vi "only_serial.vi"() -> ()   [LabVIEW 2019]
uses:
  <vilib>/Platform/TimedLoop/XDataNode/timing_clust.ctl
  <vilib>/Platform/TimedLoop/XDataNode/nitl_modes.ctl
  <vilib>/Platform/TimedLoop/XDataNode/wakeup.ctl
  <vilib>/myRIO/Instrument Drivers/Onboard IO/UART/typedef/VISA Configuration.ctl
  <vilib>/FPGAPlugInAG/myRIO-1900/niLvFpga_Open_myRIO-1900.vi
  <vilib>/rvi/interface/common/dynamic/niFpgaDynamicAddResources.vi
  <vilib>/Utility/error.llb/Error Cluster From Error Code.vi
  <vilib>/rvi/errors/niLvFpgaAdjustHostInterfaceError.vi
  <vilib>/FPGAPlugInAG/Dynamic/niLvFpga_Close_Dynamic.vi
  <vilib>/Platform/TimedLoop/XDataNode/XDataNode.xnode
  <vilib>/rvi/interface/nirviOpenFPGA/nirviOpenFPGA.xnode
  FPGA Bitfiles/capstone_FPGATarget_encoderFPGA_AeXAVEDpCcY.lvbitx
  encoder_FPGA.vi
  <vilib>/rvi/interface/nirviReadWriteControl/nirviReadWriteControl.xnode
  <vilib>/rvi/interface/nirviCloseFPGA/nirviCloseFPGA.xnode
  <vilib>/Platform/TimedLoop/XDataNode/XDNodeRunTimeDep.lvlib
  NiFpgaLv.dll
  <vilib>/rvi/interface/Simulation/niFpgaSimulationCallBeginRW.vi
  <vilib>/myRIO/Instrument Drivers/Onboard IO/UART/UART.lvlib
panel:
  in  "timed 정지":bool
  out "신중버튼 i":i32
  out "read buffer":string
  out "2번(거리)":string
  out "1번(각도)":string
  out "불리언":bool
  out "s? t:f":dbl
  in  "error in (no error)":errorcluster
  out "error out":errorcluster
  out "1or0이 들어옴":string
  out "회전수 i":i32
  in  "신중버튼":bool
  out "x > y?":bool
  in  "L_pwm":i32=3000
  out "타임아웃":i32=-1
  in  "R_pwm":i32=3000
  out "L_encoder":i32
  out "R_Encoder":i32
  out "L_이동 거리":dbl
  out "R_이동 거리":dbl
  out "mm/ms":dbl
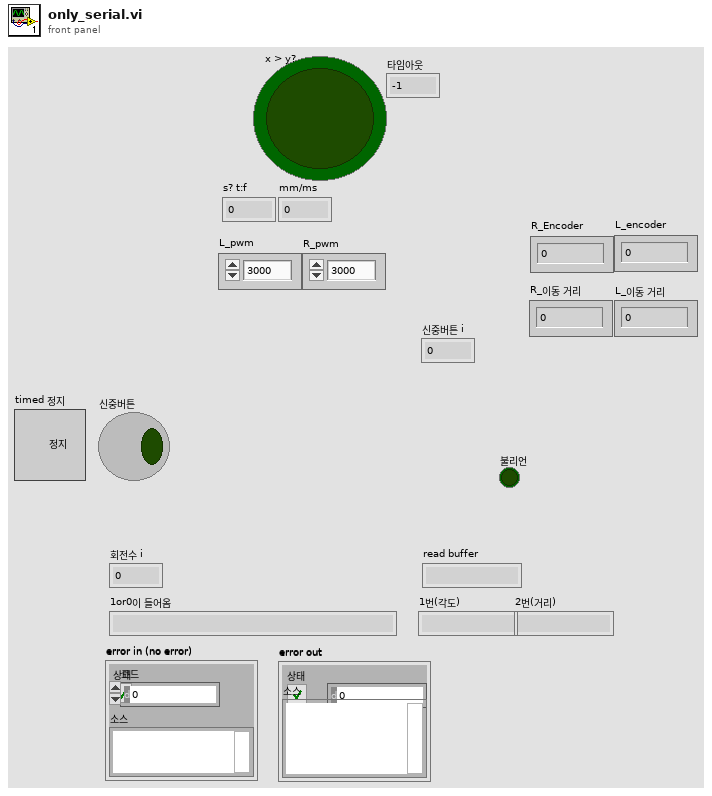
[diagram p1: front panel]
types:
  T1 = typedef "XDNodeRunTimeDep.lvlib/timing_clust.ctl" = cluster{"Expected End [f-1]":u64, "Actual End [f-1]":u64, "Finished Late? [f-1]":bool, "Expected End [i-1]":u64, "Actual End [i-1]":u64, "Finished Late? [i-1]":bool, "Expected Start [i]":u64, "Actual Start [i]":u64, "Expected Start [f]":u64, "Actual Start [f]":u64, "Source Name":string, "Structure Name":string, "Period":i64, "Deadline":i64, "Offset":i64, "Start":i64, "Priority":i32, "Timeout":i32, "Mode":T2, "Wakeup Reason":T3, "Error":errorcluster, "Source Type":string, "Secondary Source Type":string, "Global End Time":u64, "Global Start Time":u64, "Frame Duration":u64, "Iteration Duration":u64, "Assigned CPU":i32, "I/O Scan Engine Mode":u32}
  T2 = typedef "XDNodeRunTimeDep.lvlib/nitl_modes.ctl" = enum32{"No Change", "Process missed periods, maintain original phase", "Discard missed periods, maintain original phase", "Process missed periods, ignore original phase", "Discard missed periods, ignore original phase"}
  T3 = typedef "XDNodeRunTimeDep.lvlib/wakeup.ctl" = enum32{"Normal", "Aborted", "Asynchronous wakeup", "Timing source error", "Timed loop error", "Timeout"}
  T4 = typedef "UART.lvlib/VISA Configuration.ctl" = cluster{"baud rate (9600)":u32, "data bits (8)":u16, "parity (0:none)":enum16{"None", "Odd", "Even", "Mark", "Space"}, "stop bits (10: 1 bit)":u16, "flow control (0:none)":u16, "termination char\n(0xA = '\\n' = LF) ":u8, "Enable Termination\nChar (T)":bool, "timeout (10sec)":u32}
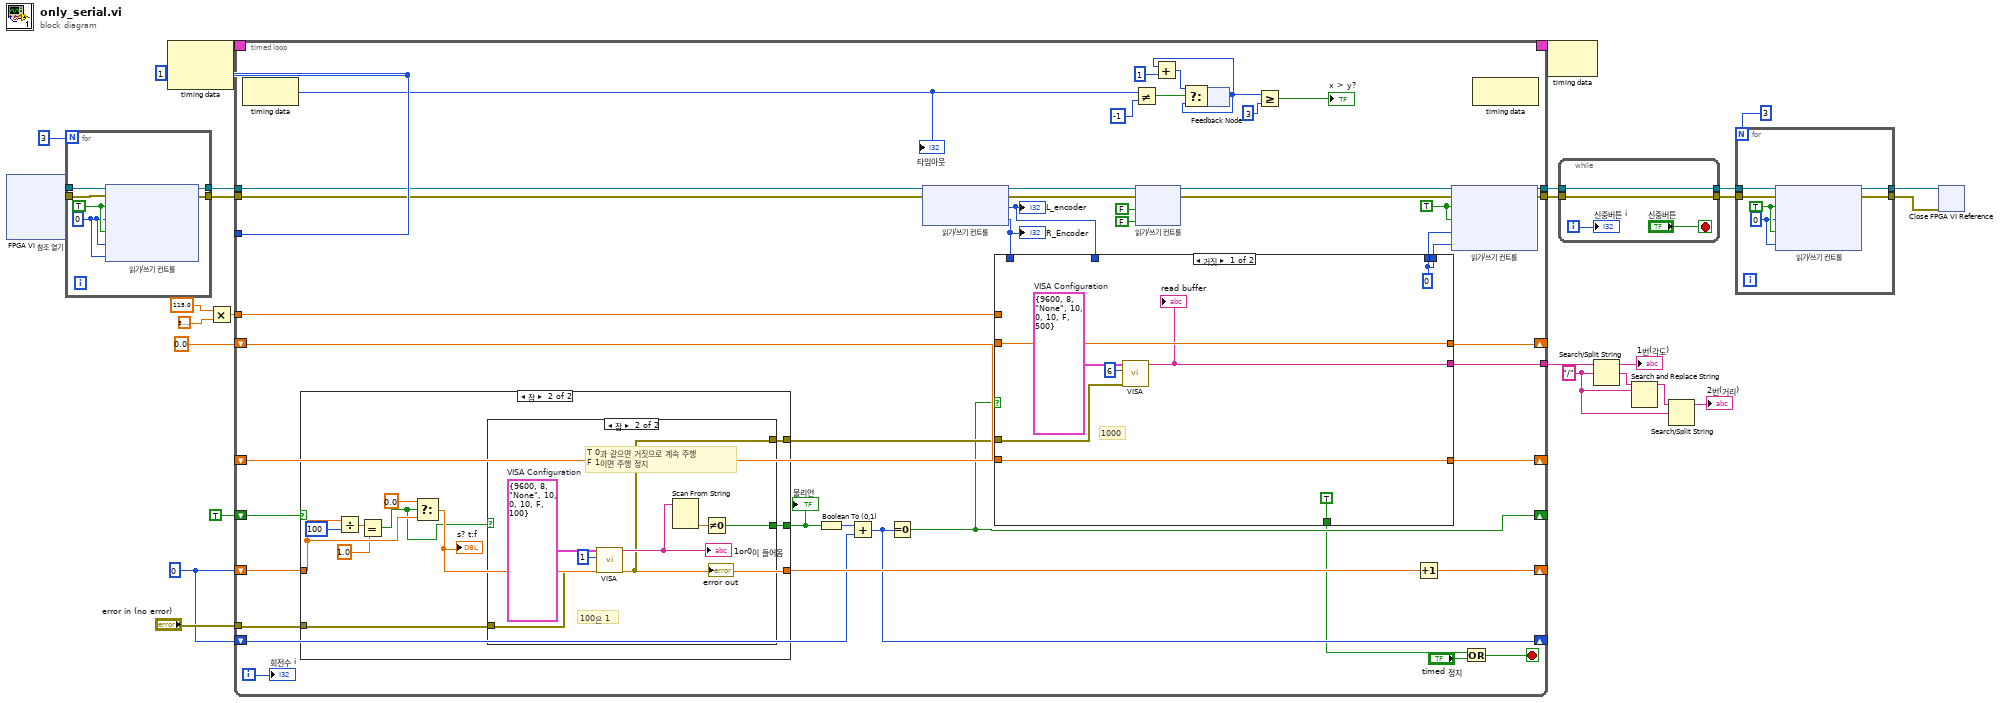
[diagram p0: block diagram]
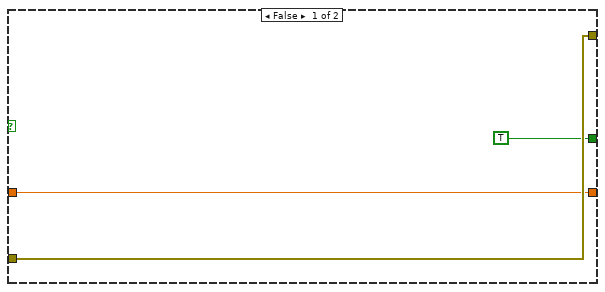
[diagram p2: hidden frame]
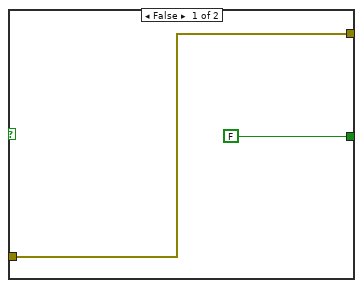
[diagram p3: hidden frame]
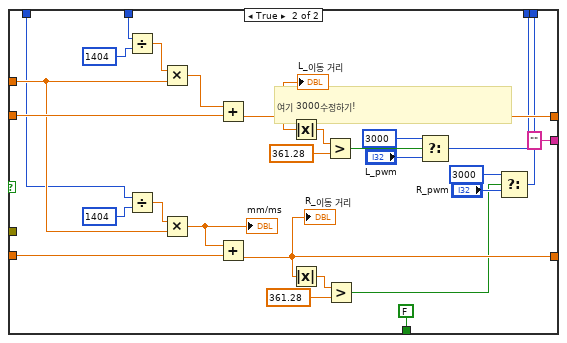
[diagram p4: hidden frame]
diagram:
  w10 = "/" ("검색 문자열/문자 (-)")
  w12 = 0
  w18 = 0.0
  w19 = i64 1 ("주기")
  n1 = xnode "FPGA VI 참조 열기"() -> ("FPGA VI 참조 출력"=w17:refnum<k20>, "에러 출력"=w16:errorcluster)  [unwired: 2 in]
  n2 = for {
    N: 3 -> [_]
    tunnel: [w34] -> w25
    tunnel: [w33] -> w24
    tunnel: w17 -> [w30]
    tunnel: w16 -> [w29]
    w31 = 0 ("pwm input(escon)")
    w32 = TRUE ("encoder reset")
    n3 = xnode "읽기/쓰기 컨트롤"("FPGA VI 참조 입력"=w30, "에러 입력"=w29, "encoder reset"=w32, "pwm input"=w31, "R_encoder reset"=w32, "R_pwm input"=w31, "직동_pwm input"=w31) -> ("FPGA VI 참조 출력"=w34:refnum<k20>, "에러 출력"=w33:errorcluster)
  }
  n4 = node-c288(w19) -> (w28:T1)  [unwired: 1 in]
  n5 = Multiply(x=115.0, y=3.141592653589793) -> (x*y=w20:dbl)
  n6 = timed-loop {
    timing: w28 -> [_]
    timing-out: [_] -> w27
    tunnel: w25 -> [w67]
    tunnel: w24 -> [w66]
    tunnel: [w70] -> w4
    tunnel: [w69] -> w1
    tunnel: w20 -> [w58]
    tunnel: w19 -> [_]
    shift-right: [w61] -> _
    shift-left: w18 -> [w59]
    shift-right: [w51] -> _
    shift-left: w18 -> [w60]
    tunnel: "error in (no error)" -> [w49]
    shift-right: [w48] -> _
    shift-left: w12 -> [w46]
    shift-right: [w42] -> _
    shift-left: w12 -> [w43]
    shift-right: [w39] -> _
    shift-left: TRUE -> [w40]
    tunnel: [w38] -> w6
    i -> [w50]
    stop <- w37 stop-if-true
    w68 = TRUE ("encoder reset")
    n7 = node-c288() -> (w79:i32)  [unwired: 1 in]
    "타임아웃" <- w79
    n8 = case shown="참" w40 {
      tunnel: w49 -> [w82 w92]
      tunnel: [w80 w90] -> w47
      tunnel: w46 -> [w80 w88]
      tunnel: [TRUE w84] -> w44
      tunnel: [w82 w83] -> w41
      frame False {
      }
      frame True {
        n9 = Divide(x=w88, y=100) -> (x/y=w87:dbl)
        n10 = Equal?(x=w87, y=1.0) -> (x = y?=w85:bool)
        n11 = Select(t=0.0, s=w85, f=w88) -> (s? t:f=w90:dbl)
        "s? t:f" <- w90
        n12 = case shown="참" w85 {
          tunnel: w92 -> [w93 w101]
          tunnel: [FALSE w100] -> w84
          tunnel: [w93 w95] -> w83
          frame False {
          }
          frame True {
            w98 = T4 {"baud rate (9600)"=9600, "data bits (8)"=8, "parity (0:none)"=enum."None", "stop bits (10: 1 bit)"=10, "flow control (0:none)"=0, "termination char\n(0xA = '\\n' = LF) "=10, "Enable Termination\nChar (T)"=FALSE, "timeout (10sec)"=100}  # VISA Configuration
            # "100은 1"
            # "T 0과 같으면 거짓으로 계속 주행\nF 1이면 주행 정지"
            n13 = call "VISA.vi"("에러 입력(에러 없음)"=w101, "바이트 카운트"=u32 1, "VISA Configuration"=w98) -> ("에러 출력"=w95:errorcluster, "read buffer"=w96:string)  [unwired: 7 in]
            "error out" <- w95
            "1or0이 들어옴" <- w96
            n14 = Scan From String(input string=w96) -> (output 1=w99:dbl)  [unwired: 4 in, 3 out]
            n15 = Not Equal To 0?(x=w99) -> (x != 0?=w100:bool)
          }
        }
      }
    }
    "불리언" <- w44
    n16 = Boolean To (0,1)(Boolean=w44) -> (0, 1=w45:i16)
    n17 = Add(x=w45, y=w43) -> (x+y=w42:i32)
    n18 = Equal To 0?(x=w42) -> (x = 0?=w39:bool)
    n19 = xnode "읽기/쓰기 컨트롤"("FPGA VI 참조 입력"=w67, "에러 입력"=w66) -> ("FPGA VI 참조 출력"=w64:refnum<k20>, "에러 출력"=w63:errorcluster, "Encoder  (4x)"=w57:i32, "R_Encoder  (4x)"=w56:i32)
    "L_encoder" <- w57
    "R_Encoder" <- w56
    n20 = case shown="거짓" w39 {
      tunnel: [w106 w136] -> w61
      tunnel: w60 -> [w107 w135]
      tunnel: w59 -> [w106 w134]
      tunnel: w58 -> [_ w133]
      tunnel: w57 -> [_ w132]
      tunnel: w56 -> [_ w131]
      tunnel: [TRUE FALSE] -> w36
      tunnel: [w109 w119] -> w53
      tunnel: [w109 w114] -> w52
      tunnel: [w107 w113] -> w51
      tunnel: w41 -> [w103 _]
      tunnel: [w102 "" ("read buffer")] -> w38
      frame False {
        w105 = T4 {"baud rate (9600)"=9600, "data bits (8)"=8, "parity (0:none)"=enum."None", "stop bits (10: 1 bit)"=10, "flow control (0:none)"=0, "termination char\n(0xA = '\\n' = LF) "=10, "Enable Termination\nChar (T)"=FALSE, "timeout (10sec)"=500}  # VISA Configuration
        w109 = 0 ("L_pwm")
        # "1000"
        n21 = call "VISA.vi"("에러 입력(에러 없음)"=w103, "바이트 카운트"=u32 6, "VISA Configuration"=w105) -> ("read buffer"=w102:string)  [unwired: 7 in, 1 out]
        "read buffer" <- w102
      }
      frame True {
        # "여기 3000수정하기!"
        n22 = Divide(x=w132, y=1404) -> (x/y=w127:dbl)
        n23 = Divide(x=w131, y=1404) -> (x/y=w122:dbl)
        n24 = Multiply(x=w127, y=w133) -> (x*y=w129:dbl)
        n25 = Multiply(x=w122, y=w133) -> (x*y=w124:dbl)
        "mm/ms" <- w124
        n26 = Add(x=w129, y=w134) -> (x+y=w136:dbl)
        "L_이동 거리" <- w136
        n27 = Add(x=w124, y=w135) -> (x+y=w113:dbl)
        "R_이동 거리" <- w113
        n28 = Absolute Value(x=w136) -> (abs(x)=w126:dbl)
        n29 = Absolute Value(x=w113) -> (abs(x)=w121:dbl)
        n30 = Greater?(x=w126, y=361.28) -> (0:w120:bool)
        n31 = Greater?(x=w121, y=361.28) -> (0:w112:bool)
        n32 = Select(t=3000, s=w120, f="L_pwm") -> (s? t:f=w119:i32)
        n33 = Select(t=3000, s=w112, f="R_pwm") -> (s? t:f=w114:i32)
      }
    }
    n34 = Not Equal?(x=w79, y=-1) -> (x != y?=w77:bool)
    n35 = xnode "읽기/쓰기 컨트롤"("FPGA VI 참조 입력"=w64, "에러 입력"=w63, "R_dir"=FALSE, "L_dir"=FALSE) -> ("FPGA VI 참조 출력"=w65:refnum<k20>, "에러 출력"=w62:errorcluster)
    n36 = feedback #1() -> (w73:u8)  [unwired: 1 in]
    n37 = Add(x=w73, y=u8 1) -> (x+y=w76:u8)
    n38 = Select(t=w76, s=w77, f=w73) -> (s? t:f=w75:u8)
    n39 = feedback-in #1(w75) -> ()
    n40 = Greater Or Equal?(x=w73, y=u8 3) -> (x >= y?=→"x > y?":bool)
    n41 = Increment(x=w47) -> (x+1=w48:dbl)
    n42 = xnode "읽기/쓰기 컨트롤"("FPGA VI 참조 입력"=w65, "에러 입력"=w62, "encoder reset"=w68, "R_encoder reset"=w68, "pwm input"=w53, "R_pwm input"=w52) -> ("FPGA VI 참조 출력"=w70:refnum<k20>, "에러 출력"=w69:errorcluster)
    n43 = Or(x=w36, y="timed 정지") -> (x .or. y?=w37:bool)
    n44 = node-c288() -> ()  [unwired: 1 in, 1 out]
    "회전수 i" <- w50
  }
  n45 = node-c288(w27) -> ()  [unwired: 1 out]
  n46 = while {
    tunnel: w4 -> [w143]
    tunnel: [w143] -> w3
    tunnel: [w142] -> w2
    tunnel: w1 -> [w142]
    i -> [w140]
    stop <- "신중버튼" stop-if-true
    "신중버튼 i" <- w140
  }
  n47 = Search/Split String(string=w6, search string/char (-)=w10) -> (substring before match=→"1번(각도)":string, match + rest of string=w9:string)  [unwired: 2 out]
  n48 = Search and Replace String(input string=w9, search string=w10) -> (result string=w8:string)  [unwired: 1 in, 8 out]
  n49 = Search/Split String(string=w8, search string/char (-)=w10) -> (substring before match=→"2번(거리)":string)  [unwired: 3 out]
  n50 = for {
    N: 3 -> [_]
    tunnel: w3 -> [w149]
    tunnel: w2 -> [w148]
    tunnel: [w145] -> w15
    tunnel: [w144] -> w14
    w146 = 0 ("pwm input(escon)")
    w147 = TRUE ("encoder reset")
    n51 = xnode "읽기/쓰기 컨트롤"("FPGA VI 참조 입력"=w149, "에러 입력"=w148, "encoder reset"=w147, "pwm input"=w146, "R_encoder reset"=w147, "R_pwm input"=w146) -> ("FPGA VI 참조 출력"=w145:refnum<k20>, "에러 출력"=w144:errorcluster)
  }
  n52 = xnode "Close FPGA VI Reference"("FPGA VI 참조 입력"=w15, "에러 입력"=w14) -> ()  [unwired: 1 out]
